vi "DAQ (SubVI).vi"(8 "error in (no error)":errorcluster) -> (0 "error out":errorcluster, 1 "Number of Disconnections":u32, 2 "Available Elements for Reading":i32, 3 "DAQ?":bool)   [LabVIEW 2017]
uses:
  <vilib>/Utility/file.llb/Write Delimited Spreadsheet (string).vi
  <vilib>/Utility/file.llb/Read Delimited Spreadsheet (string).vi
  <resource>/objmgr/ni.dex.rc
  <vilib>/Utility/file.llb/Write Delimited Spreadsheet (DBL).vi
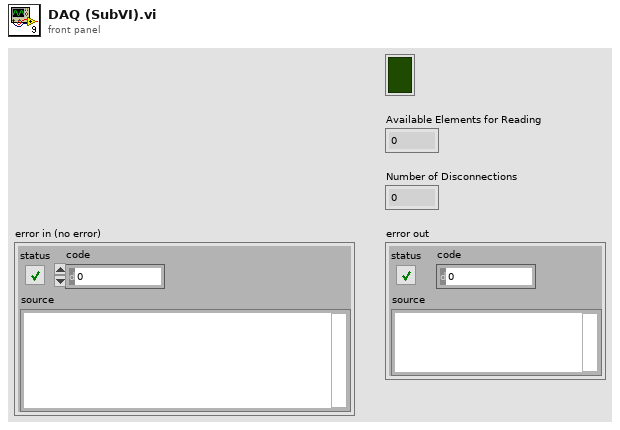
[diagram p1: front panel]
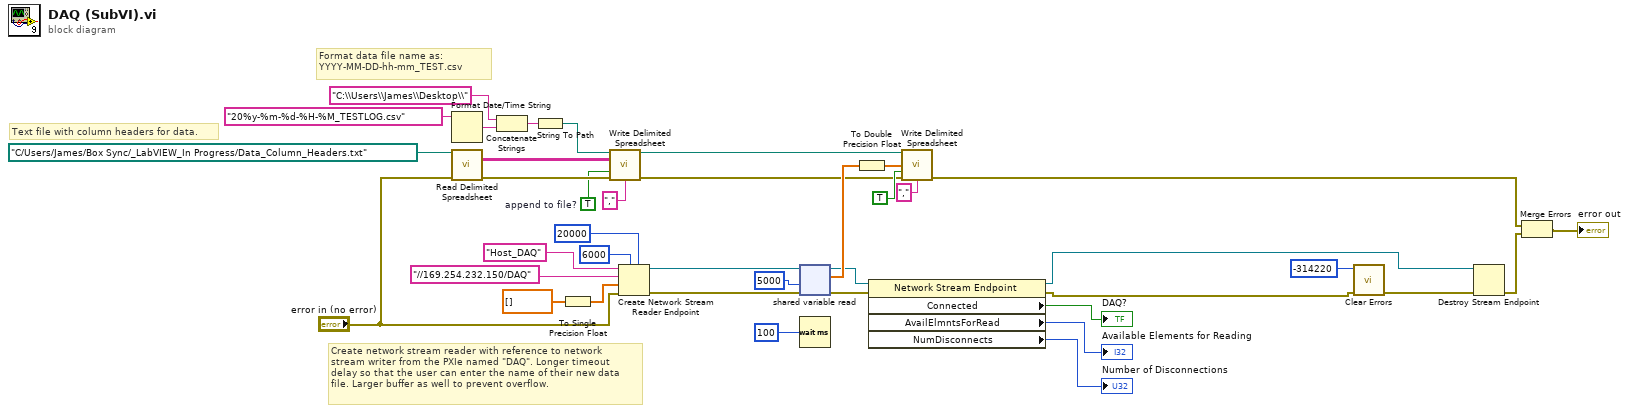
[diagram p0: block diagram]
diagram:
  w14 = TRUE  # append to file?
  # "Format data file name as:\nYYYY-MM-DD-hh-mm_TEST.csv"
  # "Create network stream reader with reference to network\nstream writer from the PXIe named \"DAQ\". Longer timeout\ndelay so that the user can enter the name of their new data\nfile. Larger buffer as well to prevent overflow."
  # "Text file with column headers for data."
  n1 = Format Date/Time String(time format string (%c)="20%y-%m-%d-%H-%M_TESTLOG.csv") -> (date/time string=w24:string)  [unwired: 2 in]
  n2 = call-poly <vilib>:"Read Delimited Spreadsheet.vi"("file path (dialog if empty)"=path "C:/Users/James/Box Sync/_LabVIEW_In Progress/Data_Column_Headers.txt", "error in (no error)"="error in (no error)") -> ("all rows"=w11:string[][], "error out"=w16:errorcluster)  [unwired: 8 in, 4 out]
  n3 = Concatenate Strings("C:\\Users\\James\\Desktop\\" ("string"), w24) -> (w22:string)
  n4 = String To Path(string=w22) -> (path=w25:path)
  n5 = To Single Precision Float(number=dbl[] []) -> (single precision float=w3:sgl[])
  n6 = call-poly <vilib>:"Write Delimited Spreadsheet.vi"("file path (dialog if empty)"=w25, "2D data"=w11, "append to file? (new file:F)"=w14, "error in (no error)"=w16, "delimiter (\\t)"=",") -> ("new file path (Not A Path if cancelled)"=w15:path, "error out"=w17:errorcluster)  [unwired: 9 in]
  n7 = Create Network Stream Reader Endpoint(5:20000 ("timeout in ms (-1)"), 7:6000 ("reader buffer size"), 8:"error in (no error)", 9:w3, 10:"//169.254.232.150/DAQ" ("writer url"), 11:"Host_DAQ" ("reader name")) -> (0:w6:errorcluster, 3:w7:refnum<k21>)  [unwired: 1 in]
  n8 = shared-variable-read(w7, w6, 5000 ("timeout ms (-1)")) -> (w29:refnum<k21>, w30:errorcluster, w35:sgl[])  [unwired: 1 out]
  n9 = Wait (ms)(milliseconds to wait=u32 100) -> ()  [unwired: 1 out]
  n10 = To Double Precision Float(number=w35) -> (double precision float=w38:dbl[])
  n11 = property class="Network Stream Endpoint"(reference=w29, error in=w30) -> (reference out=w9:refnum<k21>, error out=w39:errorcluster, "Connected"=→"DAQ?":bool, "AvailElmntsForRead"=→"Available Elements for Reading":i32, "NumDisconnects"=→"Number of Disconnections":u32)
  n12 = call-poly <vilib>:"Write Delimited Spreadsheet.vi"("file path (dialog if empty)"=w15, "1D data"=w38, "append to file? (new file:F)"=TRUE, "error in (no error)"=w17, "delimiter (\\t)"="," ("delimiter (\\t)")) -> ("error out"=w18:errorcluster)  [unwired: 9 in, 1 out]
  n13 = call <vilib>:"Clear Errors.vi"("error in (no error)"=w39, "specific error code to clear (0: all)"=-314220) -> ("error out"=w8:errorcluster)  [unwired: 4 in, 1 out]
  n14 = Destroy Stream Endpoint(8:w8, 11:w9) -> (0:w19:errorcluster)
  n15 = Merge Errors(w18, w19) -> (→"error out":errorcluster)
